vi "Lines Convert.vi"(10 "Mode":T1(ring), 11 "Lines(X,Y)":cluster{"X":dbl, "Y":dbl}={"X"=10.0, "Y"=10.0}) -> (2 "Line to Line":dbl[](array[numeric]), 3 "Lines Para":dbl[][](array[numeric]))   [LabVIEW 2015]
panel:
  out "error out":errorcluster
  in  "error in (no error)":errorcluster
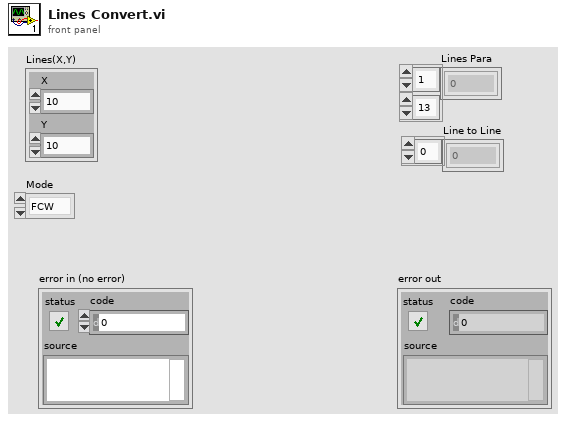
[diagram p1: front panel]
types:
  T1 = enum16{"FCW", "BSD(Right)", "BSD(Left)", "RCTA(Right)", "RCTA(Left)", "DOW(Right)", "DOW(Left)"}
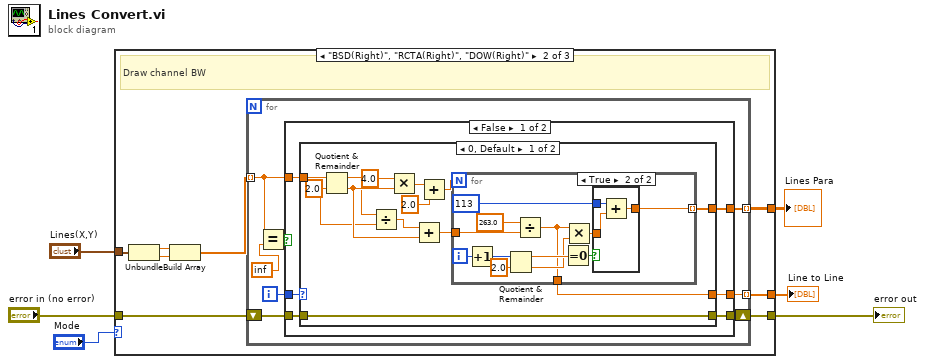
[diagram p0: block diagram]
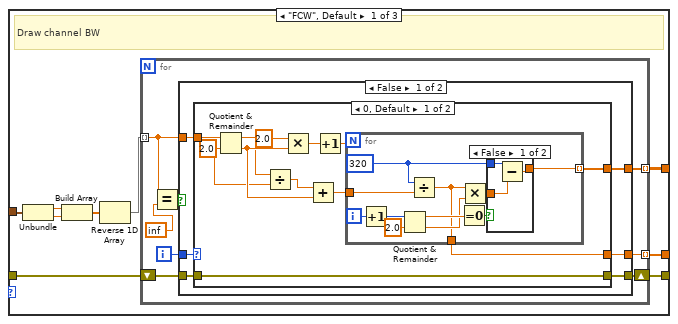
[diagram p2: hidden frame]
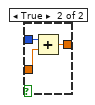
[diagram p3: hidden frame]
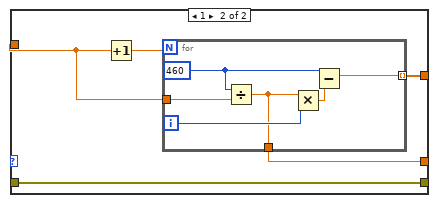
[diagram p4: hidden frame]
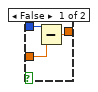
[diagram p6: hidden frame]
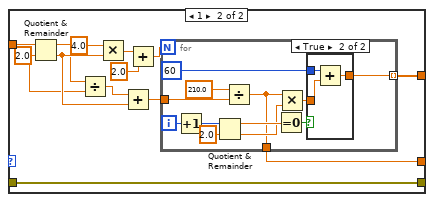
[diagram p7: hidden frame]
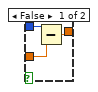
[diagram p8: hidden frame]
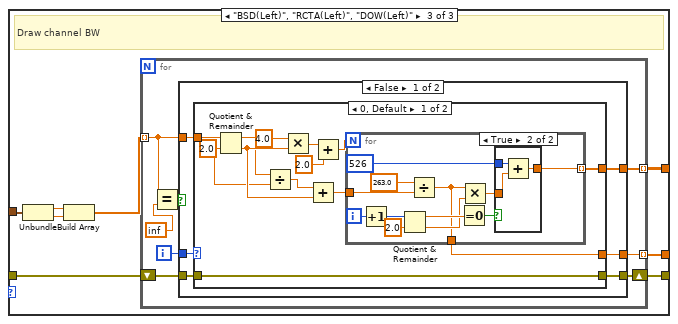
[diagram p10: hidden frame]
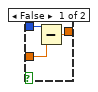
[diagram p11: hidden frame]
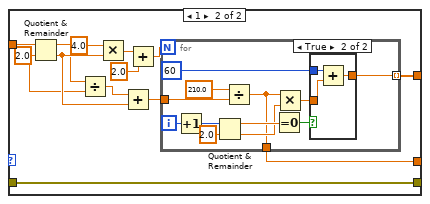
[diagram p12: hidden frame]
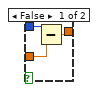
[diagram p13: hidden frame]
diagram:
  n1 = case shown="\"BSD(Right)\", \"RCTA(Right)\", \"DOW(Right)\"" "Mode" {
    tunnel: "error in (no error)" -> [w15 w78 w163]
    tunnel: [w14 w77 w162] -> w2
    tunnel: "Lines(X,Y)" -> [w13 w76 w161]
    tunnel: [w8 w72 w157] -> w4
    tunnel: [w7 w71 w156] -> w5
    frame "FCW", Default {
      # "Draw channel BW"
      n2 = Unbundle(w13) -> ("X"=w12:dbl, "Y"=w11:dbl)
      n3 = Build Array(w12, w11) -> (w10:dbl[])
      n4 = Reverse 1D Array(array=w10) -> (reversed array=w9:dbl[])
      n5 = for {
        shift-right: [w22] -> w14
        shift-left: w15 -> [w23]
        tunnel: w9 -> [w20] mode=indexing
        tunnel: [w17] -> w8 mode=indexing
        tunnel: [w16] -> w7 mode=indexing
        i -> [w21]
        n6 = Equal?(x=w20, y=inf) -> (x = y?=w19:bool)
        n7 = case shown="False" w19 {
          tunnel: w23 -> [w29 w70]
          tunnel: [w28 w70] -> w22
          tunnel: w20 -> [w27 _]
          tunnel: w21 -> [w26 _]
          tunnel: [w25 _] -> w17
          tunnel: [w24 _] -> w16
          frame False {
            n8 = case shown="0, Default" w26 {
              tunnel: w29 -> [w32 w61]
              tunnel: [w32 w61] -> w28
              tunnel: w27 -> [w33 w63]
              tunnel: [w31 w60] -> w25
              tunnel: [w30 w59] -> w24
              frame 0, Default {
                w36 = 2.0 ("y")
                n9 = Quotient & Remainder(x=w33, y=w36) -> (x-y*floor(x/y)=w35:dbl, floor(x/y)=w37:dbl)
                n10 = Divide(x=w35, y=w36) -> (x/y=w34:dbl)
                n11 = Multiply(x=2.0, y=w37) -> (x*y=w40:dbl)
                n12 = Add(x=w34, y=w37) -> (x+y=w38:dbl)
                n13 = Increment(x=w40) -> (x+1=w41:dbl)
                n14 = for {
                  N: w41 -> [_]
                  tunnel: w38 -> [w52]
                  tunnel: [w43] -> w30 mode=indexing
                  tunnel: [w42] -> w31
                  i -> [w49]
                  w44 = 320
                  n15 = Increment(x=w49) -> (x+1=w45:i32)
                  n16 = Quotient & Remainder(x=w45, y=2.0) -> (x-y*floor(x/y)=w48:dbl, floor(x/y)=w46:dbl)
                  n17 = Divide(x=w44, y=w52) -> (x/y=w42:dbl)
                  n18 = Equal To 0?(x=w48) -> (x = 0?=w47:bool)
                  n19 = Multiply(x=w42, y=w46) -> (x*y=w51:dbl)
                  n20 = case shown="False" w47 {
                    tunnel: w44 -> [w55 w58]
                    tunnel: w51 -> [w54 w57]
                    tunnel: [w53 w56] -> w43
                    frame False {
                      n21 = Subtract(x=w55, y=w54) -> (x-y=w53:dbl)
                    }
                    frame True {
                      n22 = Add(x=w58, y=w57) -> (x+y=w56:dbl)
                    }
                  }
                }
              }
              frame 1 {
                n23 = Increment(x=w63) -> (x+1=w62:dbl)
                n24 = for {
                  N: w62 -> [_]
                  tunnel: w63 -> [w69]
                  tunnel: [w65] -> w59 mode=indexing
                  tunnel: [w64] -> w60
                  i -> [w66]
                  w67 = 460
                  n25 = Divide(x=w67, y=w69) -> (x/y=w64:dbl)
                  n26 = Multiply(x=w64, y=w66) -> (x*y=w68:dbl)
                  n27 = Subtract(x=w67, y=w68) -> (x-y=w65:dbl)
                }
              }
            }
          }
          frame True {
          }
        }
      }
    }
    frame "BSD(Right)", "RCTA(Right)", "DOW(Right)" {
      # "Draw channel BW"
      n28 = Unbundle(w76) -> ("X"=w75:dbl, "Y"=w74:dbl)
      n29 = Build Array(w75, w74) -> (w73:dbl[])
      n30 = for {
        shift-right: [w85] -> w77
        shift-left: w78 -> [w86]
        tunnel: w73 -> [w83] mode=indexing
        tunnel: [w80] -> w72 mode=indexing
        tunnel: [w79] -> w71 mode=indexing
        i -> [w84]
        n31 = Equal?(x=w83, y=inf) -> (x = y?=w82:bool)
        n32 = case shown="False" w82 {
          tunnel: w86 -> [w92 w155]
          tunnel: [w91 w155] -> w85
          tunnel: w83 -> [w90 _]
          tunnel: w84 -> [w89 _]
          tunnel: [w88 _] -> w80
          tunnel: [w87 _] -> w79
          frame False {
            n33 = case shown="0, Default" w89 {
              tunnel: w92 -> [w95 w126]
              tunnel: [w95 w126] -> w91
              tunnel: w90 -> [w99 w130]
              tunnel: [w94 w125] -> w88
              tunnel: [w93 w124] -> w87
              frame 0, Default {
                w102 = 2.0 ("y")
                n34 = Quotient & Remainder(x=w99, y=w102) -> (x-y*floor(x/y)=w101:dbl, floor(x/y)=w103:dbl)
                n35 = Divide(x=w101, y=w102) -> (x/y=w100:dbl)
                n36 = Multiply(x=4.0, y=w103) -> (x*y=w98:dbl)
                n37 = Add(x=w100, y=w103) -> (x+y=w104:dbl)
                n38 = Add(x=w98, y=2.0) -> (x+y=w96:dbl)
                n39 = for {
                  N: w96 -> [_]
                  tunnel: w104 -> [w117]
                  tunnel: [w107] -> w93 mode=indexing
                  tunnel: [w106] -> w94
                  i -> [w114]
                  n40 = Increment(x=w114) -> (x+1=w110:i32)
                  n41 = Quotient & Remainder(x=w110, y=2.0) -> (x-y*floor(x/y)=w113:dbl, floor(x/y)=w111:dbl)
                  n42 = Divide(x=263.0, y=w117) -> (x/y=w106:dbl)
                  n43 = Equal To 0?(x=w113) -> (x = 0?=w112:bool)
                  n44 = Multiply(x=w106, y=w111) -> (x*y=w116:dbl)
                  n45 = case shown="True" w112 {
                    tunnel: 113 -> [w120 w123]
                    tunnel: w116 -> [w119 w122]
                    tunnel: [w118 w121] -> w107
                    frame False {
                      n46 = Subtract(x=w120, y=w119) -> (x-y=w118:dbl)
                    }
                    frame True {
                      n47 = Add(x=w123, y=w122) -> (x+y=w121:dbl)
                    }
                  }
                }
              }
              frame 1 {
                w133 = 2.0 ("y")
                n48 = Quotient & Remainder(x=w130, y=w133) -> (x-y*floor(x/y)=w132:dbl, floor(x/y)=w134:dbl)
                n49 = Divide(x=w132, y=w133) -> (x/y=w131:dbl)
                n50 = Multiply(x=4.0, y=w134) -> (x*y=w129:dbl)
                n51 = Add(x=w131, y=w134) -> (x+y=w135:dbl)
                n52 = Add(x=w129, y=2.0) -> (x+y=w127:dbl)
                n53 = for {
                  N: w127 -> [_]
                  tunnel: w135 -> [w148]
                  tunnel: [w138] -> w124 mode=indexing
                  tunnel: [w137] -> w125
                  i -> [w145]
                  n54 = Increment(x=w145) -> (x+1=w141:i32)
                  n55 = Quotient & Remainder(x=w141, y=2.0) -> (x-y*floor(x/y)=w144:dbl, floor(x/y)=w142:dbl)
                  n56 = Divide(x=210.0, y=w148) -> (x/y=w137:dbl)
                  n57 = Equal To 0?(x=w144) -> (x = 0?=w143:bool)
                  n58 = Multiply(x=w137, y=w142) -> (x*y=w147:dbl)
                  n59 = case shown="True" w143 {
                    tunnel: 60 -> [w151 w154]
                    tunnel: w147 -> [w150 w153]
                    tunnel: [w149 w152] -> w138
                    frame False {
                      n60 = Subtract(x=w151, y=w150) -> (x-y=w149:dbl)
                    }
                    frame True {
                      n61 = Add(x=w154, y=w153) -> (x+y=w152:dbl)
                    }
                  }
                }
              }
            }
          }
          frame True {
          }
        }
      }
    }
    frame "BSD(Left)", "RCTA(Left)", "DOW(Left)" {
      # "Draw channel BW"
      n62 = Unbundle(w161) -> ("X"=w160:dbl, "Y"=w159:dbl)
      n63 = Build Array(w160, w159) -> (w158:dbl[])
      n64 = for {
        shift-right: [w170] -> w162
        shift-left: w163 -> [w171]
        tunnel: w158 -> [w168] mode=indexing
        tunnel: [w165] -> w157 mode=indexing
        tunnel: [w164] -> w156 mode=indexing
        i -> [w169]
        n65 = Equal?(x=w168, y=inf) -> (x = y?=w167:bool)
        n66 = case shown="False" w167 {
          tunnel: w171 -> [w177 w240]
          tunnel: [w176 w240] -> w170
          tunnel: w168 -> [w175 _]
          tunnel: w169 -> [w174 _]
          tunnel: [w173 _] -> w165
          tunnel: [w172 _] -> w164
          frame False {
            n67 = case shown="0, Default" w174 {
              tunnel: w177 -> [w180 w211]
              tunnel: [w180 w211] -> w176
              tunnel: w175 -> [w184 w215]
              tunnel: [w179 w210] -> w173
              tunnel: [w178 w209] -> w172
              frame 0, Default {
                w187 = 2.0 ("y")
                n68 = Quotient & Remainder(x=w184, y=w187) -> (x-y*floor(x/y)=w186:dbl, floor(x/y)=w188:dbl)
                n69 = Divide(x=w186, y=w187) -> (x/y=w185:dbl)
                n70 = Multiply(x=4.0, y=w188) -> (x*y=w183:dbl)
                n71 = Add(x=w185, y=w188) -> (x+y=w189:dbl)
                n72 = Add(x=w183, y=2.0) -> (x+y=w181:dbl)
                n73 = for {
                  N: w181 -> [_]
                  tunnel: w189 -> [w202]
                  tunnel: [w192] -> w178 mode=indexing
                  tunnel: [w191] -> w179
                  i -> [w199]
                  n74 = Increment(x=w199) -> (x+1=w195:i32)
                  n75 = Quotient & Remainder(x=w195, y=2.0) -> (x-y*floor(x/y)=w198:dbl, floor(x/y)=w196:dbl)
                  n76 = Divide(x=263.0, y=w202) -> (x/y=w191:dbl)
                  n77 = Equal To 0?(x=w198) -> (x = 0?=w197:bool)
                  n78 = Multiply(x=w191, y=w196) -> (x*y=w201:dbl)
                  n79 = case shown="True" w197 {
                    tunnel: 526 -> [w205 w208]
                    tunnel: w201 -> [w204 w207]
                    tunnel: [w203 w206] -> w192
                    frame False {
                      n80 = Subtract(x=w205, y=w204) -> (x-y=w203:dbl)
                    }
                    frame True {
                      n81 = Add(x=w208, y=w207) -> (x+y=w206:dbl)
                    }
                  }
                }
              }
              frame 1 {
                w218 = 2.0 ("y")
                n82 = Quotient & Remainder(x=w215, y=w218) -> (x-y*floor(x/y)=w217:dbl, floor(x/y)=w219:dbl)
                n83 = Divide(x=w217, y=w218) -> (x/y=w216:dbl)
                n84 = Multiply(x=4.0, y=w219) -> (x*y=w214:dbl)
                n85 = Add(x=w216, y=w219) -> (x+y=w220:dbl)
                n86 = Add(x=w214, y=2.0) -> (x+y=w212:dbl)
                n87 = for {
                  N: w212 -> [_]
                  tunnel: w220 -> [w233]
                  tunnel: [w223] -> w209 mode=indexing
                  tunnel: [w222] -> w210
                  i -> [w230]
                  n88 = Increment(x=w230) -> (x+1=w226:i32)
                  n89 = Quotient & Remainder(x=w226, y=2.0) -> (x-y*floor(x/y)=w229:dbl, floor(x/y)=w227:dbl)
                  n90 = Divide(x=210.0, y=w233) -> (x/y=w222:dbl)
                  n91 = Equal To 0?(x=w229) -> (x = 0?=w228:bool)
                  n92 = Multiply(x=w222, y=w227) -> (x*y=w232:dbl)
                  n93 = case shown="True" w228 {
                    tunnel: 60 -> [w236 w239]
                    tunnel: w232 -> [w235 w238]
                    tunnel: [w234 w237] -> w223
                    frame False {
                      n94 = Subtract(x=w236, y=w235) -> (x-y=w234:dbl)
                    }
                    frame True {
                      n95 = Add(x=w239, y=w238) -> (x+y=w237:dbl)
                    }
                  }
                }
              }
            }
          }
          frame True {
          }
        }
      }
    }
  }
  "Lines Para" <- w5
  "Line to Line" <- w4
  "error out" <- w2
